vi "labview5.vi"() -> ()   [LabVIEW 2019]
uses:
  <vilib>/addons/eal4LabVIEW/eal4LabVIEW.lvlib
  <vilib>/addons/eal4LabVIEW/ApiLib/Connection control/ealApiConnect_string.vi
  <vilib>/Utility/inputDevices.llb/joystickAcquire.vi
  <vilib>/Utility/inputDevices.llb/closeJoystick.vi
panel:
  out "appended array":bool[](array[boolean])
  out "In Range? (1)":bool
  out "In Range? (2)":bool
  out "In Range? (3)":bool
  in  "condition 6":i32(ring) items=["AXIS_CONDITION_ACTIVE"=0, "AXIS_CONDITION_PARKING"=1, "AXIS_CONDITION_DEACTIVATED"=2, "AXIS_CONDITION_ACTIVE_DECOUPLED"=4, "AXIS_CONDITION_PARKING_DECOUPLED"=5, "AXIS_CONDITION_DEACTIVATED_DECOUPLED"=6, "AXIS_CONDITION_ACTIVE_PARAMETERIZATION"=8, "AXIS_CONDITION_PARKING_PARAMETERIZATION"=9, "AXIS_CONDITION_DEACTIVATED_PARAMETERIZATION"=10, "AXIS_CONDITION_ACTIVE_DECOUPLED_PARAMETERIZATION"=12, "AXIS_CONDITION_PARKING_DECOUPLED_PARAMETERIZATION"=13, "AXIS_CONDITION_DEACTIVATED_DECOUPLED_PARAMETERIZATION"=14]
  in  "slave index 6":i32
  in  "condition 5":i32(ring) items=["AXIS_CONDITION_ACTIVE"=0, "AXIS_CONDITION_PARKING"=1, "AXIS_CONDITION_DEACTIVATED"=2, "AXIS_CONDITION_ACTIVE_DECOUPLED"=4, "AXIS_CONDITION_PARKING_DECOUPLED"=5, "AXIS_CONDITION_DEACTIVATED_DECOUPLED"=6, "AXIS_CONDITION_ACTIVE_PARAMETERIZATION"=8, "AXIS_CONDITION_PARKING_PARAMETERIZATION"=9, "AXIS_CONDITION_DEACTIVATED_PARAMETERIZATION"=10, "AXIS_CONDITION_ACTIVE_DECOUPLED_PARAMETERIZATION"=12, "AXIS_CONDITION_PARKING_DECOUPLED_PARAMETERIZATION"=13, "AXIS_CONDITION_DEACTIVATED_DECOUPLED_PARAMETERIZATION"=14]
  in  "slave index 5":i32
  in  "condition 4":i32(ring) items=["AXIS_CONDITION_ACTIVE"=0, "AXIS_CONDITION_PARKING"=1, "AXIS_CONDITION_DEACTIVATED"=2, "AXIS_CONDITION_ACTIVE_DECOUPLED"=4, "AXIS_CONDITION_PARKING_DECOUPLED"=5, "AXIS_CONDITION_DEACTIVATED_DECOUPLED"=6, "AXIS_CONDITION_ACTIVE_PARAMETERIZATION"=8, "AXIS_CONDITION_PARKING_PARAMETERIZATION"=9, "AXIS_CONDITION_DEACTIVATED_PARAMETERIZATION"=10, "AXIS_CONDITION_ACTIVE_DECOUPLED_PARAMETERIZATION"=12, "AXIS_CONDITION_PARKING_DECOUPLED_PARAMETERIZATION"=13, "AXIS_CONDITION_DEACTIVATED_DECOUPLED_PARAMETERIZATION"=14]
  in  "slave index 4":i32
  out "RPM Motor 1":dbl
  out "RPM Motor 2":dbl
  out "RPM Motor 3":dbl
  in  "stop":bool
  out "return value":dbl[](array[numeric])
  out "Iteration counter":i32
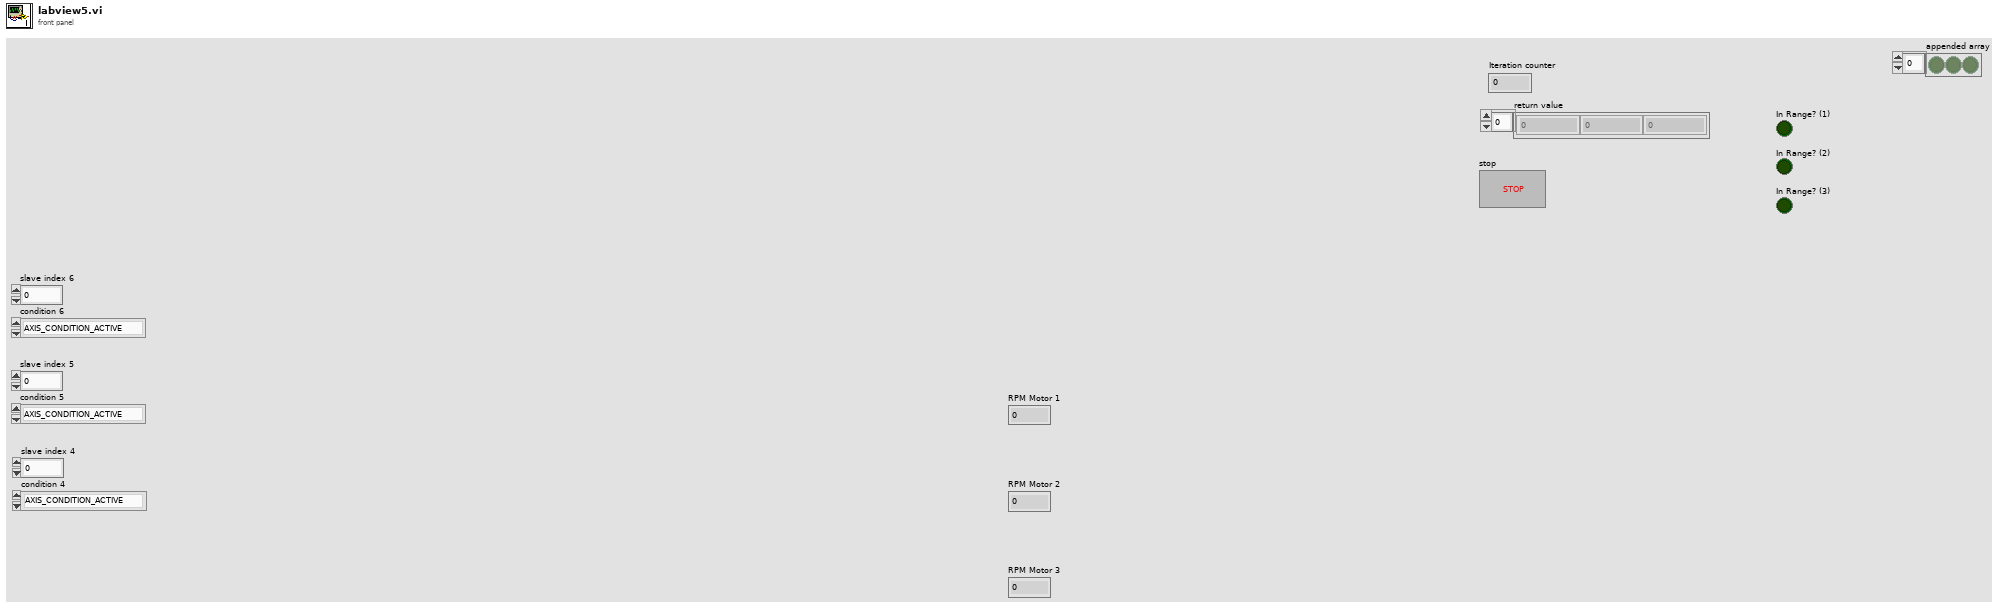
[diagram p1: front panel]
types:
  T1 = cluster{"Velocity":dbl, "Acceleration":dbl, "Deceleration":dbl, "Jerk":dbl}
  T2 = cluster{"X axis":i32, "Y axis":i32, "Z axis":i32, "X axis rotation":i32, "Y axis rotation":i32, "Z axis rotation":i32, "U axis":i32, "V axis":i32}
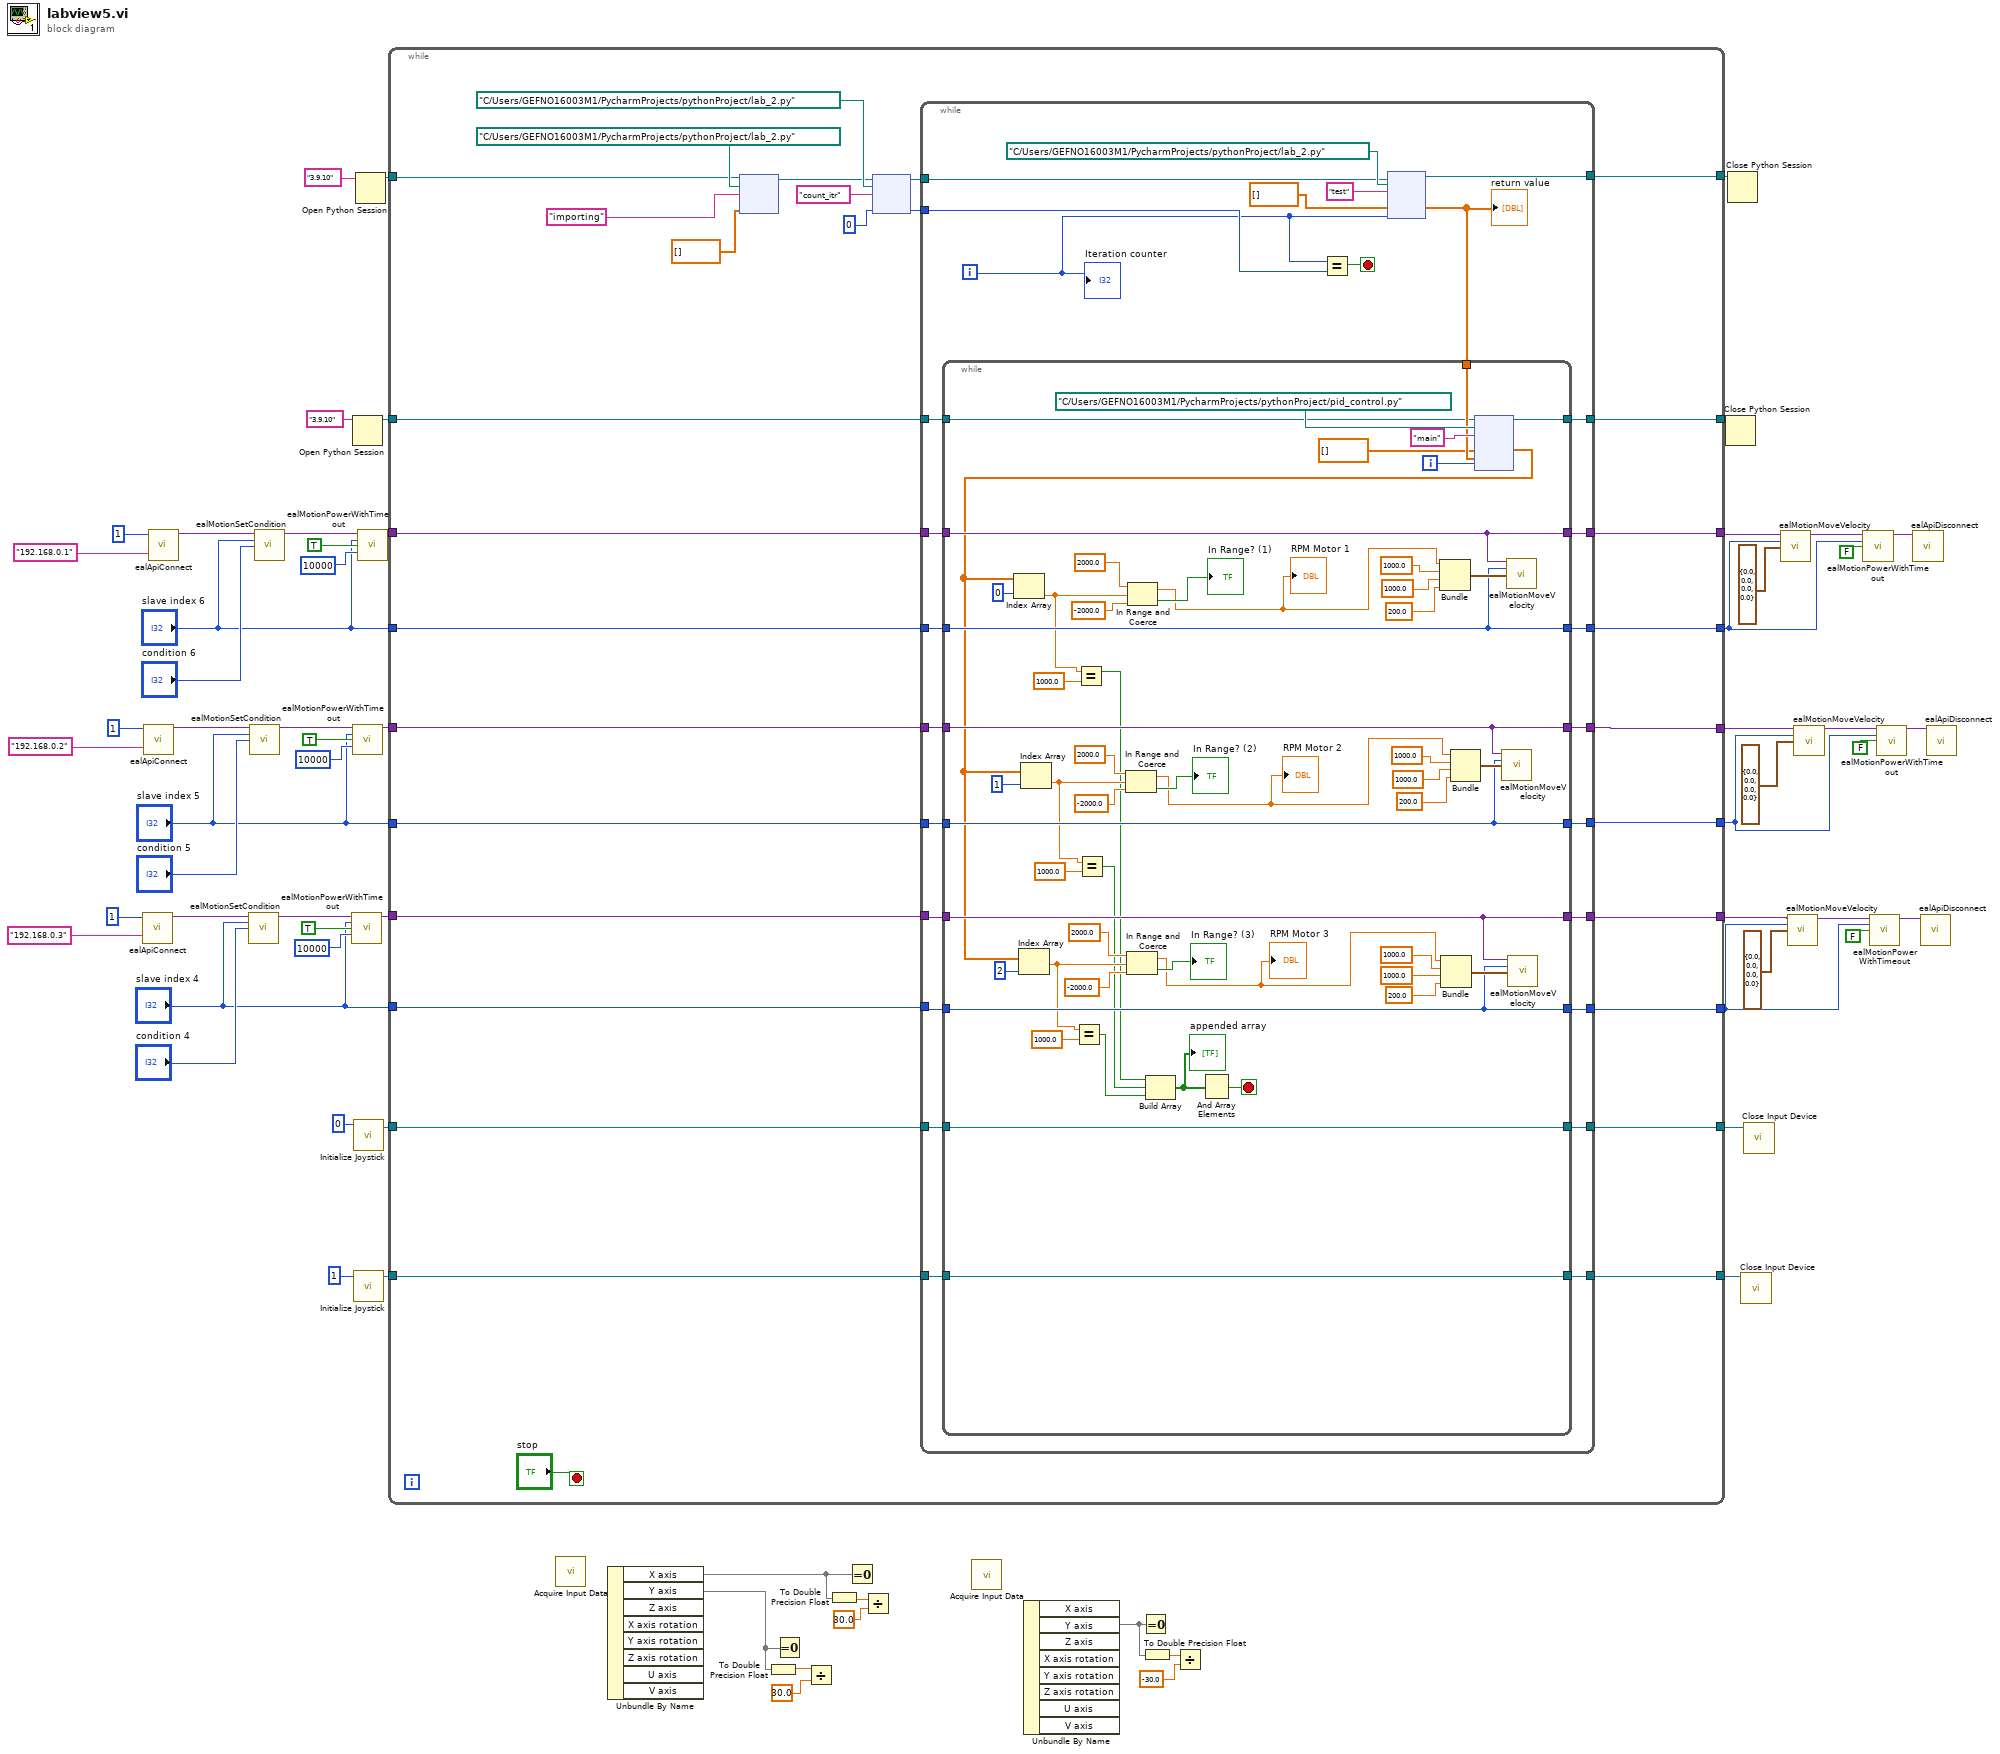
[diagram p0: block diagram]
diagram:
  n1 = call-poly <vilib>:"ealApiConnect.vi"("maximum no of axes"=1, "ip address"="192.168.0.3") -> ("connection out"=w54:variant)  [unwired: 12 in, 1 out]
  n2 = call-poly <vilib>:"ealApiConnect.vi"("maximum no of axes"=1, "ip address"="192.168.0.2") -> ("connection out"=w47:variant)  [unwired: 12 in, 1 out]
  n3 = call-poly <vilib>:"ealApiConnect.vi"("maximum no of axes"=1, "ip address"="192.168.0.1") -> ("connection out"=w40:variant)  [unwired: 12 in, 1 out]
  n4 = call <vilib>:"ealMotionSetCondition.vi"("connection in"=w54, "slave index"="slave index 4", "condition"="condition 4") -> ("connection out"=w53:variant)  [unwired: 11 in, 1 out]
  n5 = call <vilib>:"ealMotionSetCondition.vi"("connection in"=w47, "slave index"="slave index 5", "condition"="condition 5") -> ("connection out"=w46:variant)  [unwired: 11 in, 1 out]
  n6 = call <vilib>:"ealMotionSetCondition.vi"("connection in"=w40, "slave index"="slave index 6", "condition"="condition 6") -> ("connection out"=w39:variant)  [unwired: 11 in, 1 out]
  n7 = call <vilib>:"ealMotionPowerWithTimeout.vi"("connection in"=w53, "slave index"="slave index 4", "value"=TRUE, "timeout"=10000) -> ("connection out"=w33:variant)  [unwired: 10 in, 1 out]
  n8 = Open Python Session(python version="3.9.10" ("Python version")) -> (session out=w21:refnum<k35>)  [unwired: 2 in, 1 out]
  n9 = call <vilib>:"ealMotionPowerWithTimeout.vi"("connection in"=w46, "slave index"="slave index 5", "value"=TRUE, "timeout"=10000) -> ("connection out"=w34:variant)  [unwired: 10 in, 1 out]
  n10 = call <vilib>:"Initialize Joystick.vi"("device index"=0) -> ("device ID"=w15:refnum<k1>)  [unwired: 9 in, 1 out]
  n11 = call <vilib>:"Initialize Joystick.vi"("device index"=1) -> ("device ID"=w14:refnum<k1>)  [unwired: 9 in, 1 out]
  n12 = Open Python Session(python version="3.9.10" ("Python version")) -> (session out=w24:refnum<k35>)  [unwired: 2 in, 1 out]
  n13 = call <vilib>:"ealMotionPowerWithTimeout.vi"("connection in"=w39, "slave index"="slave index 6", "value"=TRUE, "timeout"=10000) -> ("connection out"=w35:variant)  [unwired: 10 in, 1 out]
  n14 = while {
    tunnel: w35 -> [w88]
    tunnel: w34 -> [w87]
    tunnel: w33 -> [w86]
    tunnel: [w85] -> w32
    tunnel: [w84] -> w31
    tunnel: "slave index 6" -> [w83]
    tunnel: "slave index 5" -> [w82]
    tunnel: [w81] -> w28
    tunnel: [w74] -> w27
    tunnel: "slave index 4" -> [w80]
    tunnel: w24 -> [w79]
    tunnel: [w78] -> w23
    tunnel: w21 -> [w77]
    tunnel: [w76] -> w20
    tunnel: [w75] -> w19
    tunnel: [w73] -> w18
    tunnel: w15 -> [w72]
    tunnel: w14 -> [w71]
    tunnel: [w70] -> w13
    tunnel: [w69] -> w12
    stop <- "stop" stop-if-true
    n15 = node(w79, path "C:/Users/GEFNO16003M1/PycharmProjects/pythonProject/lab_2.py" ("module path"), "importing" ("function name"), dbl[] []) -> (w93:refnum<k35>)  [unwired: 2 in, 3 out]
    n16 = node(w93, path "C:/Users/GEFNO16003M1/PycharmProjects/pythonProject/lab_2.py" ("module path"), "count_itr" ("function name"), 0) -> (w92:refnum<k35>, w90:i32)  [unwired: 1 in, 3 out]
    n17 = while {
      tunnel: [w119] -> w78
      tunnel: w92 -> [w122]
      tunnel: w90 -> [w120]
      tunnel: w88 -> [w117]
      tunnel: w87 -> [w106]
      tunnel: w86 -> [w116]
      tunnel: [w108] -> w85
      tunnel: [w109] -> w84
      tunnel: w83 -> [w107]
      tunnel: w82 -> [w105]
      tunnel: [w110] -> w81
      tunnel: w80 -> [w112]
      tunnel: w77 -> [w104]
      tunnel: [w114] -> w76
      tunnel: [w113] -> w75
      tunnel: [w111] -> w74
      tunnel: [w103] -> w73
      tunnel: w72 -> [w102]
      tunnel: w71 -> [w101]
      tunnel: [w100] -> w70
      tunnel: [w99] -> w69
      i -> [w115]
      stop <- w123 stop-if-true
      n18 = Equal?(x=w115, y=w120) -> (x = y?=w123:bool)
      n19 = node(w122, path "C:/Users/GEFNO16003M1/PycharmProjects/pythonProject/lab_2.py" ("module path"), "test" ("function name"), dbl[] [], w115) -> (w119:refnum<k35>, w118:dbl[])  [unwired: 2 in, 3 out]
      "return value" <- w118
      n20 = while {
        tunnel: w118 -> [w177]
        tunnel: w117 -> [w149]
        tunnel: w116 -> [w151]
        tunnel: [w151] -> w114
        tunnel: [w150] -> w113
        tunnel: w112 -> [w150]
        tunnel: [w147] -> w111
        tunnel: [w146] -> w110
        tunnel: [w148] -> w109
        tunnel: [w149] -> w108
        tunnel: w107 -> [w148]
        tunnel: w106 -> [w147]
        tunnel: w105 -> [w146]
        tunnel: w104 -> [w145]
        tunnel: [w144] -> w103
        tunnel: w102 -> [w127]
        tunnel: w101 -> [w126]
        tunnel: [w127] -> w100
        tunnel: [w126] -> w99
        i -> [w143]
        stop <- w141 stop-if-true
        n21 = node(w145, path "C:/Users/GEFNO16003M1/PycharmProjects/pythonProject/pid_control.py" ("module path"), "main" ("function name"), dbl[] [], w177, w143) -> (w144:refnum<k35>, w142:dbl[])  [unwired: 3 in, 3 out]
        n22 = Index Array(array=w142, index=0) -> (element=w137:dbl)
        n23 = Index Array(array=w142, index=2) -> (element=w135:dbl)
        n24 = Index Array(array=w142, index=1) -> (element=w136:dbl)
        n25 = Equal?(x=w135, y=1000.0) -> (x = y?=w132:bool)
        n26 = Equal?(x=w137, y=1000.0) -> (x = y?=w134:bool)
        n27 = Equal?(x=w136, y=1000.0) -> (x = y?=w133:bool)
        n28 = In Range and Coerce(upper limit=2000.0, x=w136, lower limit=-2000.0) -> (coerced(x)=w129:dbl, In Range?=→"In Range? (2)":bool)
        "RPM Motor 2" <- w129
        n29 = In Range and Coerce(upper limit=2000.0, x=w135, lower limit=-2000.0) -> (coerced(x)=w128:dbl, In Range?=→"In Range? (3)":bool)
        "RPM Motor 3" <- w128
        n30 = In Range and Coerce(upper limit=2000.0, x=w137, lower limit=-2000.0) -> (coerced(x)=w130:dbl, In Range?=→"In Range? (1)":bool)
        "RPM Motor 1" <- w130
        n31 = Build Array(w134, w133, w132) -> (w131:bool[])
        "appended array" <- w131
        n32 = And Array Elements(Boolean array=w131) -> (logical AND=w141:bool)
        n33 = Bundle("upper limit"=w130, 1000.0, 1000.0, 200.0) -> (w161:cluster{"upper limit":dbl, dbl, dbl, dbl})  [unwired: 1 in]
        n34 = Bundle("upper limit"=w128, 1000.0, 1000.0, 200.0) -> (w171:cluster{"upper limit":dbl, dbl, dbl, dbl})  [unwired: 1 in]
        n35 = Bundle("upper limit"=w129, 1000.0, 1000.0, 200.0) -> (w166:cluster{"upper limit":dbl, dbl, dbl, dbl})  [unwired: 1 in]
        n36 = call <vilib>:"ealMotionMoveVelocity.vi"("connection in"=w147, "slave index"=w146, "parameters set"=w166) -> ()  [unwired: 11 in, 2 out]
        n37 = call <vilib>:"ealMotionMoveVelocity.vi"("connection in"=w149, "slave index"=w148, "parameters set"=w161) -> ()  [unwired: 11 in, 2 out]
        n38 = call <vilib>:"ealMotionMoveVelocity.vi"("connection in"=w151, "slave index"=w150, "parameters set"=w171) -> ()  [unwired: 11 in, 2 out]
      }
      "Iteration counter" <- w115
    }
  }
  n39 = call-poly <vilib>:"Acquire Input Data.vi"() -> ()  [unwired: 15 in, 5 out]
  n40 = Unbundle By Name() -> (w11:T2, "X axis"=w10, "Y axis"=w9)  [unwired: 6 out]
  n41 = To Double Precision Float(number=w9) -> (double precision float=w5:dbl)
  n42 = Equal To 0?(x=w9) -> ()  [unwired: 1 out]
  n43 = Divide(x=w5, y=30.0) -> ()  [unwired: 1 out]
  n44 = To Double Precision Float(number=w10) -> (double precision float=w8:dbl)
  n45 = Equal To 0?(x=w10) -> ()  [unwired: 1 out]
  n46 = Divide(x=w8, y=30.0) -> ()  [unwired: 1 out]
  n47 = call-poly <vilib>:"Acquire Input Data.vi"() -> ()  [unwired: 15 in, 5 out]
  n48 = Unbundle By Name() -> (w4:T2, "Y axis"=w2)  [unwired: 7 out]
  n49 = Equal To 0?(x=w2) -> ()  [unwired: 1 out]
  n50 = To Double Precision Float(number=w2) -> (double precision float=w3:dbl)
  n51 = Divide(x=w3, y=-30.0) -> ()  [unwired: 1 out]
  n52 = Close Python Session(session in=w18) -> ()  [unwired: 1 in, 1 out]
  n53 = Close Python Session(session in=w23) -> ()  [unwired: 1 in, 1 out]
  n54 = call-poly <vilib>:"Close Input Device.vi"("device ID"=w12) -> ()  [unwired: 9 in, 1 out]
  n55 = call-poly <vilib>:"Close Input Device.vi"("device ID"=w13) -> ()  [unwired: 9 in, 1 out]
  n56 = call <vilib>:"ealMotionMoveVelocity.vi"("connection in"=w32, "slave index"=w31, "parameters set"=T1 {"Velocity"=0.0, "Acceleration"=0.0, "Deceleration"=0.0, "Jerk"=0.0}) -> ("connection out"=w59:variant)  [unwired: 11 in, 1 out]
  n57 = call <vilib>:"ealMotionMoveVelocity.vi"("connection in"=w20, "slave index"=w19, "parameters set"=T1 {"Velocity"=0.0, "Acceleration"=0.0, "Deceleration"=0.0, "Jerk"=0.0}) -> ("connection out"=w67:variant)  [unwired: 11 in, 1 out]
  n58 = call <vilib>:"ealMotionMoveVelocity.vi"("connection in"=w27, "slave index"=w28, "parameters set"=T1 {"Velocity"=0.0, "Acceleration"=0.0, "Deceleration"=0.0, "Jerk"=0.0}) -> ("connection out"=w63:variant)  [unwired: 11 in, 1 out]
  n59 = call <vilib>:"ealMotionPowerWithTimeout.vi"("connection in"=w59, "slave index"=w31, "value"=FALSE) -> ("connection out"=w60:variant)  [unwired: 11 in, 1 out]
  n60 = call <vilib>:"ealMotionPowerWithTimeout.vi"("connection in"=w67, "slave index"=w19, "value"=FALSE) -> ("connection out"=w68:variant)  [unwired: 11 in, 1 out]
  n61 = call <vilib>:"ealMotionPowerWithTimeout.vi"("connection in"=w63, "slave index"=w28, "value"=FALSE) -> ("connection out"=w64:variant)  [unwired: 11 in, 1 out]
  n62 = call <vilib>:"ealApiDisconnect.vi"("connection in"=w60) -> ()  [unwired: 14 in, 1 out]
  n63 = call <vilib>:"ealApiDisconnect.vi"("connection in"=w68) -> ()  [unwired: 14 in, 1 out]
  n64 = call <vilib>:"ealApiDisconnect.vi"("connection in"=w64) -> ()  [unwired: 14 in, 1 out]
